vi "PUT X Input Channel.vi"(0 "X Input Channel":string) -> ()   [LabVIEW 2013]
uses:
  Action.ctl
  Channel FGV Selector.ctl
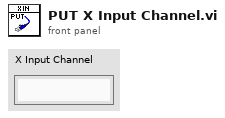
[diagram p1: front panel]
types:
  T1 = typedef "Channel FGV Selector.ctl" = enum16{"Division Input", "Sum Input", "Z Output", "Z Input", "Y Output", "Y Input", "X Output", "X Input"}
  T2 = typedef "Action.ctl" = enum16{"GET", "PUT", "DELETE"}
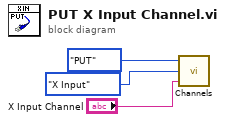
[diagram p0: block diagram]
diagram:
  n1 = call "Channels.vi"("Input"="X Input Channel", "Channel FGV Selector"=Channel_FGV_Selector."X Input", "Action"=Action."PUT") -> ()  [unwired: 1 out]
